vi "MovCorrFuncs 0.1.vi"(7 "Boundary":dbl, 8 "error in (no error)":errorcluster, 9 "MovCorrFunc":T4(ring), 10 "LUT1":cluster{u16, u16}(slide)={0, 4095} caption="Slide" scale=0.0..4095.0, 11 "Image":T2(plugin-control)) -> (0 "error out":errorcluster, 2 "Reference Rectangles":i16[][](array[numeric]), 3 "Reference Screen":T2(plugin-control))   [LabVIEW 2017]
uses:
  <vilib>/vision/Image Controls.llb/IMAQ Image.ctl
panel:
  in  "LUT 2":cluster{i16, i16}(slide)={0, 4095} scale=0.0..4095.0
  in  "LUT":cluster{i16, i16}(slide)={0, 4095} scale=0.0..4095.0
  out "Lines":T1(array[cluster]) {"End Point"."Y" format="%.2f"; "End Point"."X" format="%.2f"; "Start Point"."Y" format="%.2f"; "Start Point"."X" format="%.2f"}
  out "Number of Matches Returned":i32
  out "got copy":bool=TRUE
  out "upper":u16
  out "lower":u16
  out "Number of Particles":i32
  out "Mean Value":sgl format="%.2f"
  out "Histogram Graph":T3 {"Incremental Value" format="%.2f"; "Starting Value" format="%.2f"}
  out "temp copy":T2
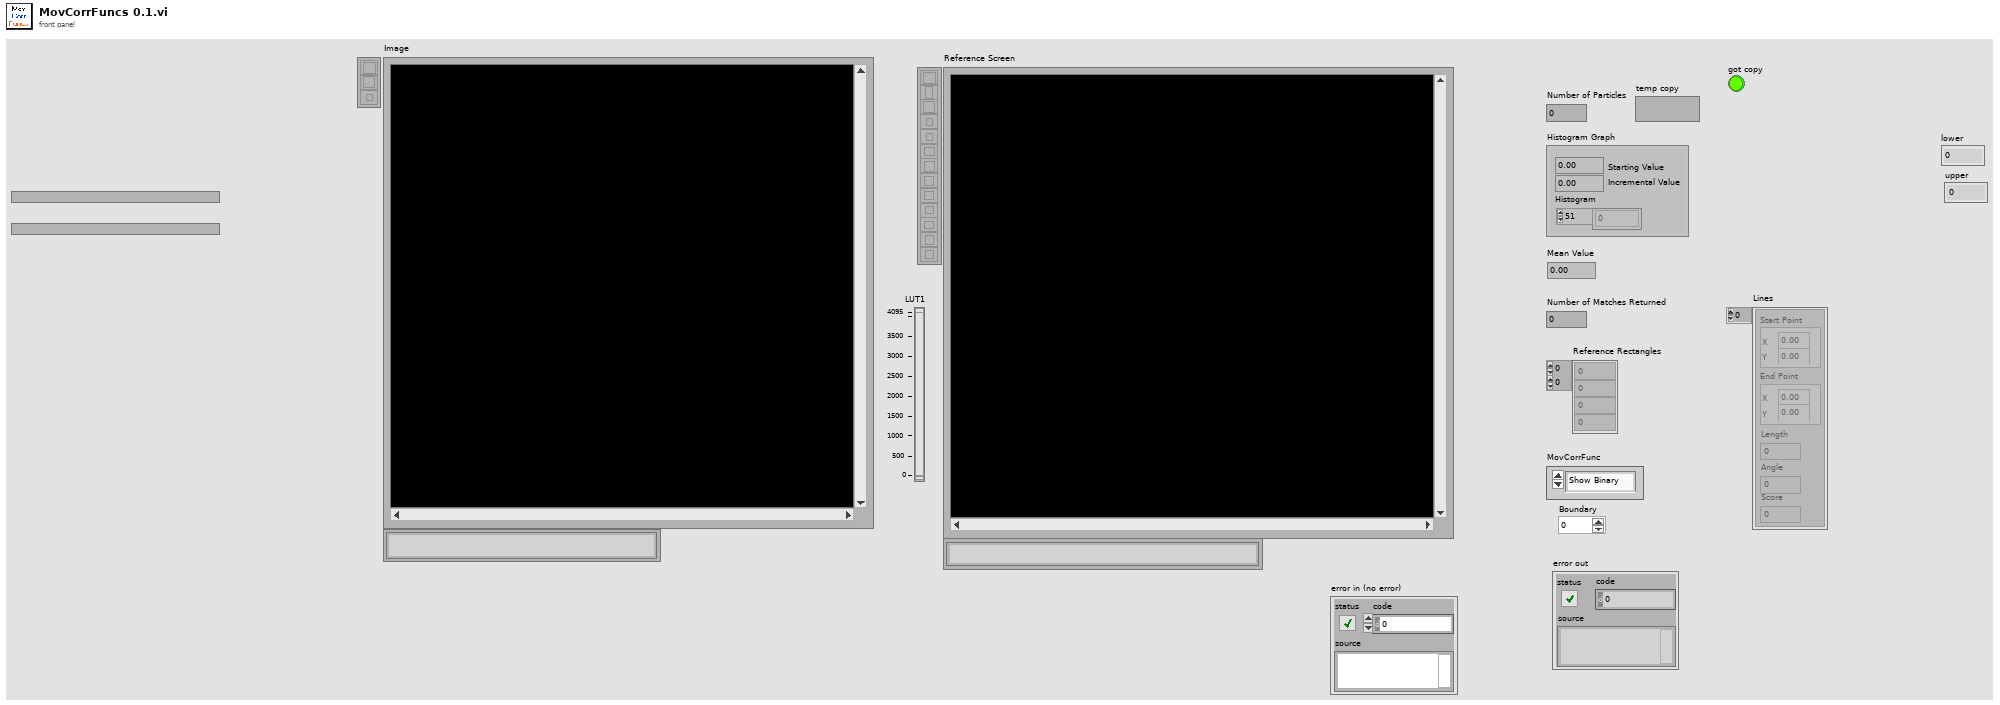
[diagram p1: front panel]
types:
  T1 = cluster{"Start Point":cluster{"X":sgl, "Y":sgl}, "End Point":cluster{"X":sgl, "Y":sgl}, "Length":dbl, "Angle":dbl, "Score":dbl}[]
  T2 = typedef "IMAQ Image.ctl" = refnum<image>
  T3 = cluster{"Starting Value":sgl, "Incremental Value":sgl, "Histogram":u32[]}
  T4 = enum16{"Show Binary", "Show Dendrite", "Find Lines"}
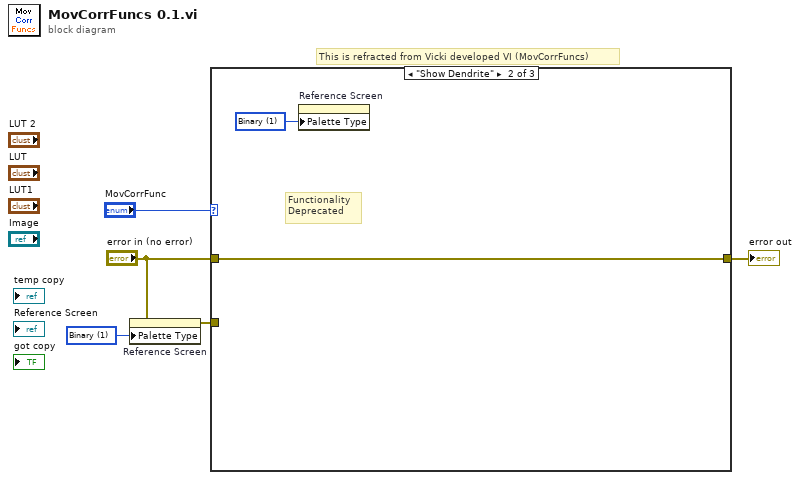
[diagram p0: block diagram]
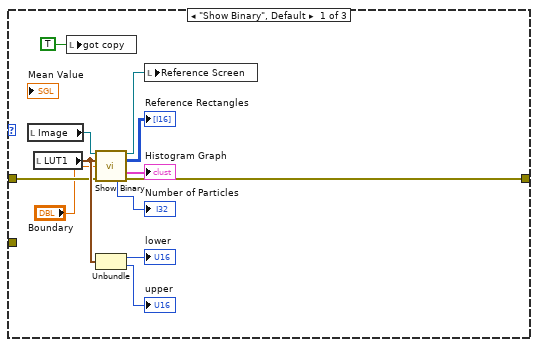
[diagram p2: hidden frame]
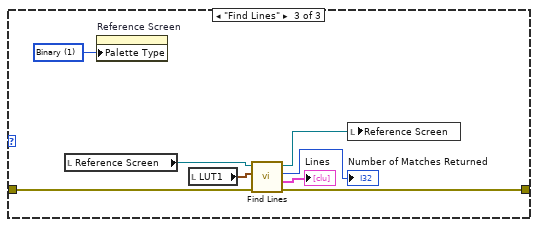
[diagram p3: hidden frame]
diagram:
  w3 = u32 1 items=["Grayscale", "Binary", "Gradient", "Rainbow", "Temperature", "User Defined"] ("Palette:Palette Type")
  # "This is refracted from Vicki developed VI (MovCorrFuncs)"
  n1 = property on="Reference Screen" class="ImageControl"(error in="error in (no error)", "Palette Type"=w3) -> (error out=w1:errorcluster)  [unwired: 1 in, 1 out]
  n2 = case shown="\"Show Dendrite\"" "MovCorrFunc" {
    tunnel: "error in (no error)" -> [w8 w18 w21]
    tunnel: [w7 w18 w20] -> w4
    tunnel: w1 -> [_ _ _]
    frame "Show Binary", Default {
      n3 = local read "Image"() -> (w12:T2)
      n4 = local read "LUT1"() -> (w9:cluster{u16, u16})
      n5 = local write "got copy"(TRUE) -> ()
      n6 = call "Show Binary.vi"("Input Image"=w12, "LUT1"=w9, "Boundary"="Boundary", "error in (no error)"=w8) -> ("Binary Image"=w10:T2, "Reference Rectangles"=→"Reference Rectangles":i16[][], "Histogram Graph"=→"Histogram Graph":T3, "Number of Particles"=→"Number of Particles":i32, "error out"=w7:errorcluster)  [unwired: 7 in]
      n7 = Unbundle(w9) -> (→"lower":u16, →"upper":u16)
      n8 = local write "Reference Screen"(w10) -> ()
    }
    frame "Show Dendrite" {
      w19 = u32 1 items=["Grayscale", "Binary", "Gradient", "Rainbow", "Temperature", "User Defined"] ("Palette:Palette Type")
      # "Functionality \nDeprecated"
      n9 = property on="Reference Screen" class="ImageControl"("Palette Type"=w19) -> ()  [unwired: 2 in, 2 out]
    }
    frame "Find Lines" {
      w25 = u32 1 items=["Grayscale", "Binary", "Gradient", "Rainbow", "Temperature", "User Defined"] ("Palette:Palette Type")
      n10 = local read "Reference Screen"() -> (w27:T2)
      n11 = property on="Reference Screen" class="ImageControl"("Palette Type"=w25) -> ()  [unwired: 2 in, 2 out]
      n12 = local read "LUT1"() -> (w26:cluster{u16, u16})
      n13 = call "Find Lines.vi"("error in (no error)"=w21, "LUT"=w26, "Image In"=w27) -> ("error out"=w20:errorcluster, "Lines"=→"Lines":T1, "Number of Matches Returned"=→"Number of Matches Returned":i32, "Image Out"=w24:T2)  [unwired: 5 in]
      n14 = local write "Reference Screen"(w24) -> ()
    }
  }
  "error out" <- w4
